vi "LN2 Extern Befuellung Warnung.vi"(0 "Date and Time":refnum<vi>, 5 "Rezept":refnum<vi>, 7 "LN2 Warnung":refnum<vi>, 11 "error in (no error)":errorcluster caption="Fehler (Eingang, kein Fehler)", 13 "Aktion":T1) -> (4 "Externe LN2 Warnung":string, 15 "error out":errorcluster caption="Fehler (Ausgang)")   [LabVIEW 2020, in "Erweiterte Konfig.lvlib"]
uses:
  Erweiterte Konfig.lvlib
  Aktion LN2 Extern Befuellung Warnung.ctl
  Anlagenuebersicht/VisBx Anzeige/Aktion FGV Ventile manuell schalten Crio.ctl
  cRIO/PC/Kommunikation mit cRIO.lvlib
  Anlagenuebersicht/VisBx Anzeige/Anlagenuebersicht.lvlib
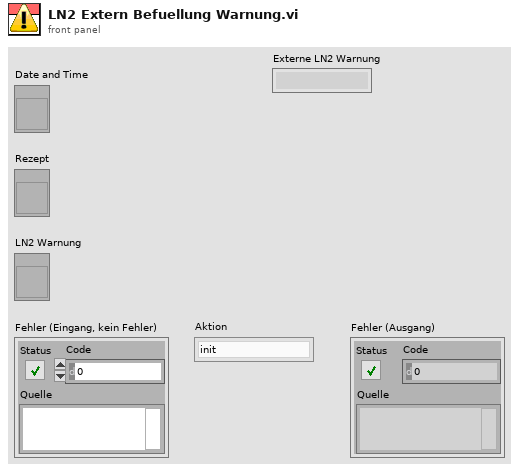
[diagram p1: front panel]
types:
  T1 = typedef "Erweiterte Konfig.lvlib/Aktion LN2 Extern Befuellung Warnung.ctl" = enum16{"init", "blinken", "Warnungen ausgeben"}
  T2 = typedef "Anlagenuebersicht.lvlib/Aktion FGV Ventile manuell schalten Crio.ctl" = enum16{"lesen", "Ventile schalten", "Testbetrieb aktiv", "Testbetrieb inaktiv", "Anzeige Ventilstellung"}
  T3 = typedef "Verwaltung - cRIO.lvlib/Digital Ausgaenge 32-63.ctl" = cluster{"O32: Messgaspumpe EIN":bool, "O33: (Umgebungsluftpumpe)":bool, "O34: (Kondensatpumpe GK)":bool, "O35: Klima/Lüfter EIN":bool, "O36: Versorgung Heizungen":bool, "O37: Versorgung Heizungen":bool, "O38: (Gaskühler EIN (Freigabe))":bool, "O39: Störung FAS LP":bool, "O40: (Heizung Filterblock)":bool, "O41: Heizung HL zu FT-IR":bool, "O42: Heizung HL Extern SP1":bool, "O43: Heizung HL Extern SP2":bool, "O44: Heizung Reserve":bool, "O45: Heizung Reserve":bool, "O46: Statusbeleuchtung grün":bool, "O47: Statusbeleuchtung rot":bool}
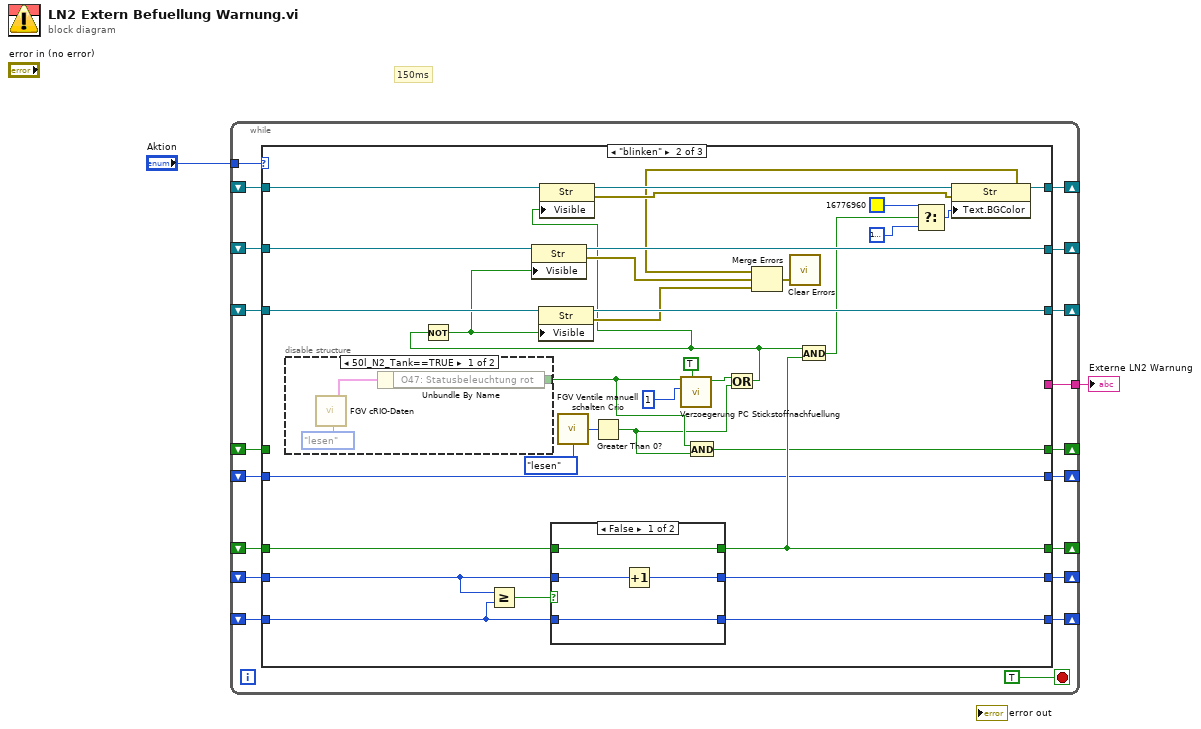
[diagram p0: block diagram]
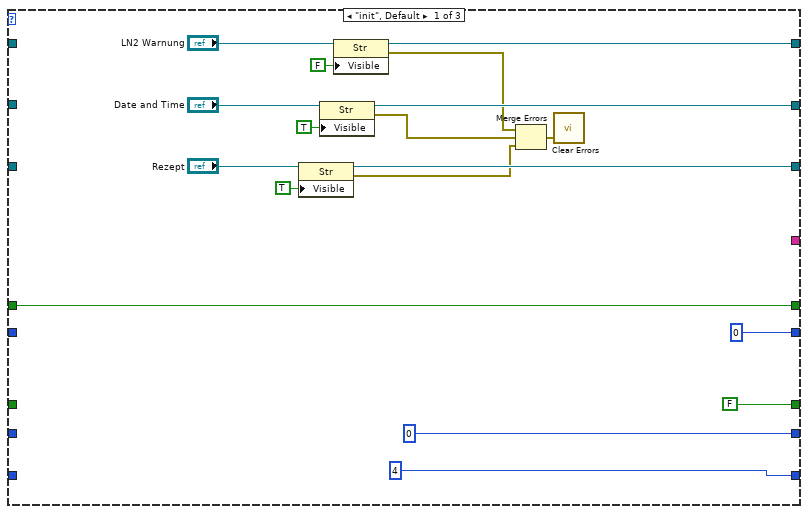
[diagram p2: hidden frame]
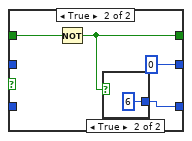
[diagram p4: hidden frame]
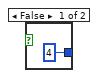
[diagram p5: hidden frame]
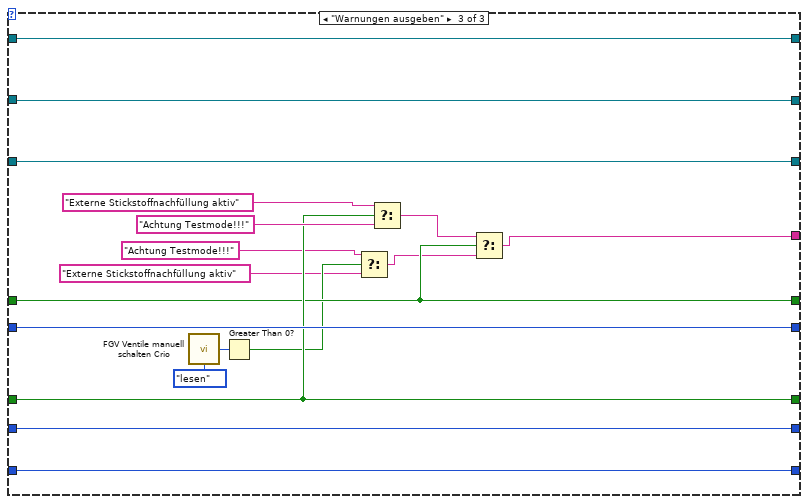
[diagram p6: hidden frame]
diagram:
  # "150ms"
  n1 = while {
    tunnel: "Aktion" -> [w20]
    shift-right: [w17] -> _
    shift-left: _ -> [w14]
    shift-right: [w18] -> _
    shift-left: _ -> [w15]
    shift-right: [w19] -> _
    shift-left: _ -> [w16]
    shift-right: [w13] -> _
    shift-left: _ -> [w12]
    shift-right: [w11] -> _
    shift-left: _ -> [w10]
    shift-right: [w9] -> _
    shift-left: _ -> [w8]
    shift-right: [w7] -> _
    shift-left: _ -> [w6]
    tunnel: [w5] -> w1
    shift-right: [w4] -> _
    shift-left: _ -> [w3]
    stop <- TRUE stop-if-true
    n2 = case shown="\"blinken\"" w20 {
      tunnel: [w33 w56 w104] -> w19
      tunnel: [w32 w62 w103] -> w18
      tunnel: [w31 w61 w102] -> w17
      tunnel: w16 -> [_ w65 w104]
      tunnel: w15 -> [_ w73 w103]
      tunnel: w14 -> [_ w72 w102]
      tunnel: [0 w71 w100] -> w13
      tunnel: w12 -> [_ w70 w100]
      tunnel: [FALSE w64 w96] -> w11
      tunnel: w10 -> [_ w68 w96]
      tunnel: [4 w67 w99] -> w9
      tunnel: w8 -> [_ w66 w99]
      tunnel: [0 w46 w101] -> w7
      tunnel: w6 -> [_ w46 w101]
      tunnel: [_ _ w87] -> w5
      tunnel: [w22 w42 w92] -> w4
      tunnel: w3 -> [w22 _ w92]
      frame "init", Default {
        n3 = property class="Str"(reference="Rezept", "Visible"=TRUE ("Sichtbar")) -> (reference out=w31:refnum<vi>, error out=w27:errorcluster)  [unwired: 1 in]
        n4 = property class="Str"(reference="Date and Time", "Visible"=TRUE ("Sichtbar")) -> (reference out=w32:refnum<vi>, error out=w28:errorcluster)  [unwired: 1 in]
        n5 = property class="Str"(reference="LN2 Warnung", "Visible"=FALSE ("Sichtbar")) -> (reference out=w33:refnum<vi>, error out=w29:errorcluster)  [unwired: 1 in]
        n6 = Merge Errors(w29, w28, w27) -> (w30:errorcluster)
        n7 = call <vilib>:"Clear Errors.vi"("error in (no error)"=w30) -> ()  [unwired: 5 in, 2 out]
      }
      frame "blinken" {
        n8 = disable-structure shown="50l_N2_Tank==TRUE" {
          disable-tunnel: [w76 _] -> w43
          frame condition #0 {
            n9 = call "FGV cRIO-Daten.vi"("Aktion"=enum16{"lesen", "schreiben"}."lesen") -> ("DO 32-63"=w74:T3)  [unwired: 9 in, 9 out]
            n10 = Unbundle By Name(w74) -> ("O47: Statusbeleuchtung rot"=w76:bool)
          }
          frame condition #1 (active) {
          }
        }
        n11 = Greater Or Equal?(x=w70, y=w66) -> (x >= y?=w69:bool)
        n12 = case shown="False" w69 {
          tunnel: w70 -> [w80 _]
          tunnel: [w77 0] -> w71
          tunnel: [w79 w81] -> w64
          tunnel: w68 -> [w79 w83]
          tunnel: w66 -> [w78 _]
          tunnel: [w78 w82] -> w67
          frame False {
            n13 = Increment(x=w80) -> (x+1=w77:i32)
          }
          frame True {
            n14 = Not(x=w83) -> (.not. x?=w81:bool)
            n15 = case shown="True" w81 {
              tunnel: [4 6] -> w82
              frame False {
              }
              frame True {
              }
            }
          }
        }
        n16 = call "FGV Ventile manuell schalten Crio.vi"("Aktion"=Aktion_FGV_Ventile_manuell_schalten_Crio."lesen") -> ("Betrieb"=w44:u16)  [unwired: 11 in, 3 out]
        n17 = Greater Than 0?(x=w44) -> (x > 0?=w40:bool)
        n18 = call "Verzoegerung PC Stickstoffnachfuellung.vi"("Abfallverzögerung?"=TRUE, "min"=u16 1, "Startsignal"=w43) -> ("Zeit abgelaufen?"=w49:bool)  [unwired: 7 in, 1 out]
        n19 = And(x=w43, y=w40) -> (x .and. y?=w42:bool)
        n20 = Or(x=w49, y=w40) -> (x .or. y?=w41:bool)
        n21 = Not(x=w41) -> (.not. x?=w60:bool)
        n22 = property class="Str"(reference=w73, "Visible"=w60) -> (reference out=w62:refnum<vi>, error out=w59:errorcluster)  [unwired: 1 in]
        n23 = property class="Str"(reference=w72, "Visible"=w60) -> (reference out=w61:refnum<vi>, error out=w58:errorcluster)  [unwired: 1 in]
        n24 = property class="Str"(reference=w65, "Visible"=w41) -> (reference out=w63:refnum<vi>, error out=w51:errorcluster)  [unwired: 1 in]
        n25 = And(x=w41, y=w64) -> (x .and. y?=w53:bool)
        n26 = Select(t=u32 16776960, s=w53, f=u32 16777226) -> (s? t:f=w52:u32)
        n27 = property class="Str"(reference=w63, error in=w51, "Text.BGColor"=w52) -> (reference out=w56:refnum<vi>, error out=w50:errorcluster)
        n28 = Merge Errors(w50, w59, w58) -> (w57:errorcluster)
        n29 = call <vilib>:"Clear Errors.vi"("error in (no error)"=w57) -> ()  [unwired: 5 in, 2 out]
      }
      frame "Warnungen ausgeben" {
        n30 = call "FGV Ventile manuell schalten Crio.vi"("Aktion"=Aktion_FGV_Ventile_manuell_schalten_Crio."lesen") -> ("Betrieb"=w95:u16)  [unwired: 11 in, 3 out]
        n31 = Greater Than 0?(x=w95) -> (x > 0?=w91:bool)
        n32 = Select(t="Achtung Testmode!!!" ("Externe LN2 Warnung"), s=w91, f="Externe Stickstoffnachfüllung aktiv" ("Externe LN2 Warnung")) -> (s? t:f=w88:string)
        n33 = Select(t="Externe Stickstoffnachfüllung aktiv" ("Externe LN2 Warnung"), s=w96, f="Achtung Testmode!!!" ("Externe LN2 Warnung")) -> (s? t:f=w93:string)
        n34 = Select(t=w93, s=w92, f=w88) -> (s? t:f=w87:string)
      }
    }
  }
  "Externe LN2 Warnung" <- w1
